vi "ACK with Horizontal Position.vi"(8 "error in (no error)":errorcluster, 9 "Horizontal position, degrees":dbl, 11 "MotionComm in":refnum<class "MotionComm.lvclass">) -> (0 "error out":errorcluster, 3 "MotionComm out":refnum<class "MotionComm.lvclass">)   [LabVIEW 2019, in "MotionComm.lvclass"]
uses:
  MotionComm.lvclass
  MotionComm.lvclass/MotionComm.ctl
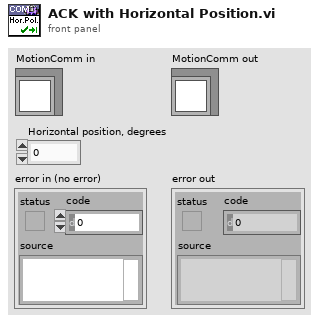
[diagram p1: front panel]
types:
  T1 = typedef "MessageQue.lvlib/MessageQue.ctl" = refnum<queue>
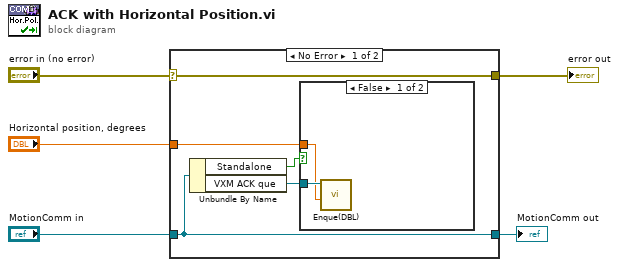
[diagram p0: block diagram]
diagram:
  n1 = case shown="No Error" "error in (no error)" {
    selector: "error in (no error)" -> [w10 w14]
    tunnel: [w10 w14] -> w4
    tunnel: [w9 w13] -> w2
    tunnel: "MotionComm in" -> [w9 w13]
    tunnel: "Horizontal position, degrees" -> [w6 _]
    frame No Error {
      n2 = Unbundle By Name(w9) -> ("Standalone"=w7:bool, "VXM ACK que"=w8:T1)
      n3 = case shown="False" w7 {
        tunnel: w8 -> [w12 _]
        tunnel: w6 -> [w11 _]
        frame False {
          n4 = call "Enque(DBL).vi"("Message Payload DBL Numeric"=w11, "Message que"=w12) -> ()  [unwired: 8 in, 2 out]
        }
        frame True {
          # "do not send ack message, \nthere's no entity to ACK to."
        }
      }
    }
    frame Error {
    }
  }
  "error out" <- w4
  "MotionComm out" <- w2
